vi "FG UDP Base.vi"(1 "FG Action (Read)":T1, 2 "UDP Base in":T2) -> (0 "UDP Base out":T2)   [LabVIEW 2009]
uses:
  UDP Lib/UDP Base.ctl
  UDP Lib/UDP Socket Params.ctl
  cRIO/Functional Global Variables/Actions for FG's.ctl
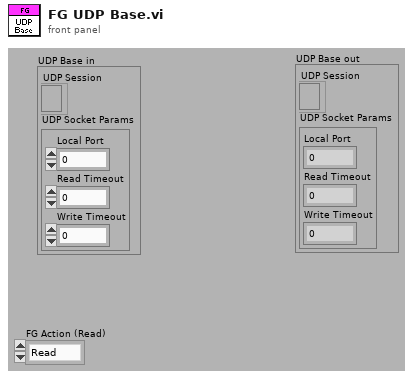
[diagram p1: front panel]
types:
  T1 = typedef "Actions for FG's.ctl" = enum16{"Read", "Write"}
  T2 = typedef "UDP Base.ctl" = cluster{"UDP Session":refnum<k16>, "UDP Socket Params":T3}
  T3 = typedef "UDP Socket Params.ctl" = cluster{"Local Port":u16, "Read Timeout":i32, "Write Timeout":i32}
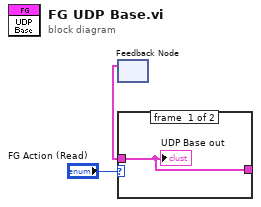
[diagram p0: block diagram]
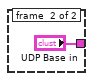
[diagram p2: hidden frame]
diagram:
  n1 = feedback #1() -> (w1:T2)  [unwired: 1 in]
  n2 = case shown="\"Read\", Default" "FG Action (Read)" {
    tunnel: w1 -> [w4 _]
    tunnel: [w4 "UDP Base in"] -> w2
    frame #0 {
      "UDP Base out" <- w4
    }
    frame #1 {
    }
  }
